vi "Write stopped event.vi"(8 "error in (no error)":errorcluster, 10 "stopped event":refnum<user-event>, 11 "ConfigurableActor in":refnum<class "ConfigurableActor.lvclass">) -> (0 "error out":errorcluster, 3 "ConfigurableActor out":refnum<class "ConfigurableActor.lvclass">)   [LabVIEW 2014, in "ConfigurableActor.lvclass"]
uses:
  ConfigurableActor.lvclass
  ConfigurableActor.lvclass/ConfigurableActor.ctl
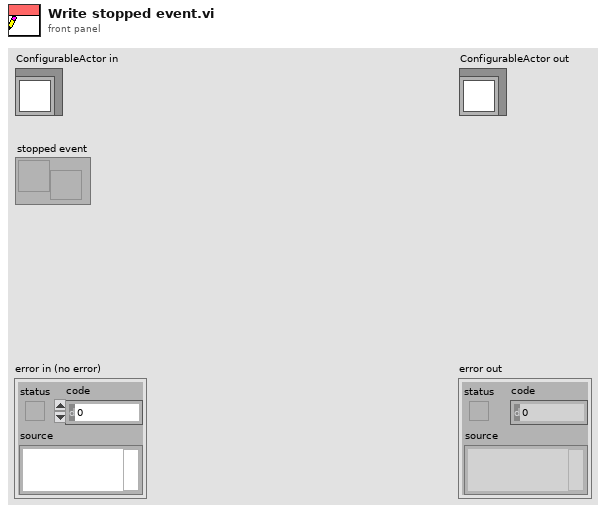
[diagram p1: front panel]
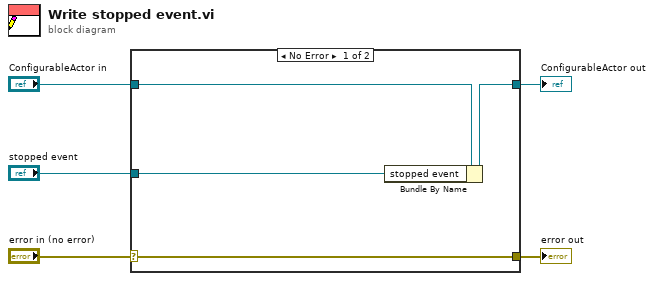
[diagram p0: block diagram]
diagram:
  n1 = case shown="No Error" "error in (no error)" {
    selector: "error in (no error)" -> [w9 w10]
    tunnel: [w9 w10] -> w4
    tunnel: [w6 w11] -> w2
    tunnel: "ConfigurableActor in" -> [w8 w11]
    tunnel: "stopped event" -> [w7 _]
    frame No Error {
      n2 = Bundle By Name(cluster=w8, "stopped event"=w7) -> (w6:refnum<class "ConfigurableActor.lvclass">)
    }
    frame Error {
    }
  }
  "error out" <- w4
  "ConfigurableActor out" <- w2
